vi "MainPhaseSpaceTracking.vi"() -> ()   [LabVIEW 2017]
uses:
  libowlsock.dll
panel:
  out "concatenated string":string
  in  "Button  Or UDP Sync":bool
  out "InvertVisualFbk":bool
  out "Imposed Time":i32
  out "Obj Initial Pos":dbl
  in  "Data Saveing Dir":string="Z:\\Toma_S\\DataProofs\\PhaseSpace\\"
  out "Shoulder":bool
  out "Elbow":bool
  out "refnum out":refnum<file>
  out "Data Filename":path
  out "Block":i32
  out "trial":u8
  out "Recording Switch":bool caption="Off       On"
  in  "Recording State":bool
  in  "UDP Sender Ip address":string="127.0.0.1"
  in  "ZeroTime":u32
  in  "ZeroFrame":i32
  out "Loop Time":u32
  out "Elapsed time (msec)":dbl
  out "Markers":dbl[](array[numeric])
  out "Frame Number":dbl
  in  "server address":string="192.168.0.101"
  out "connected\nto server?":bool
  out "Wrist":bool
  out "object":bool
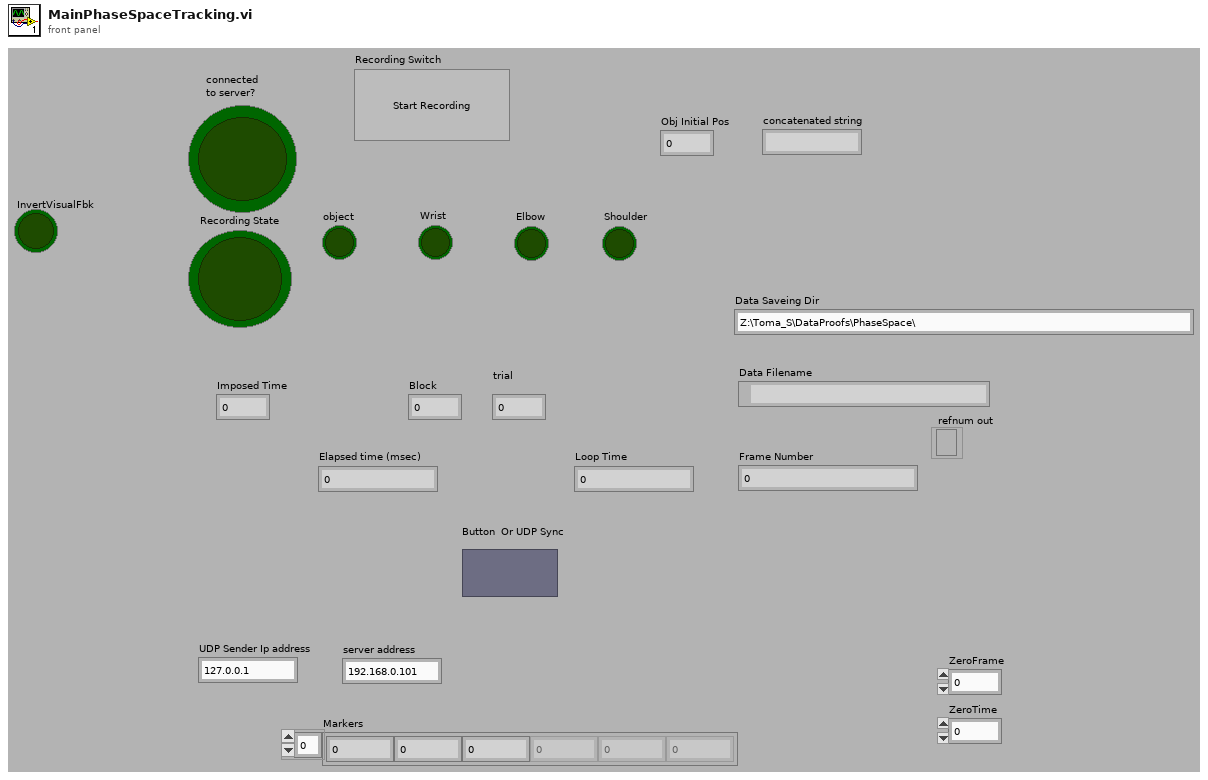
[diagram p1: front panel]
types:
  T1 = enum16{"open", "replace", "create", "open or create", "replace or create", "replace or create with confirmation"}
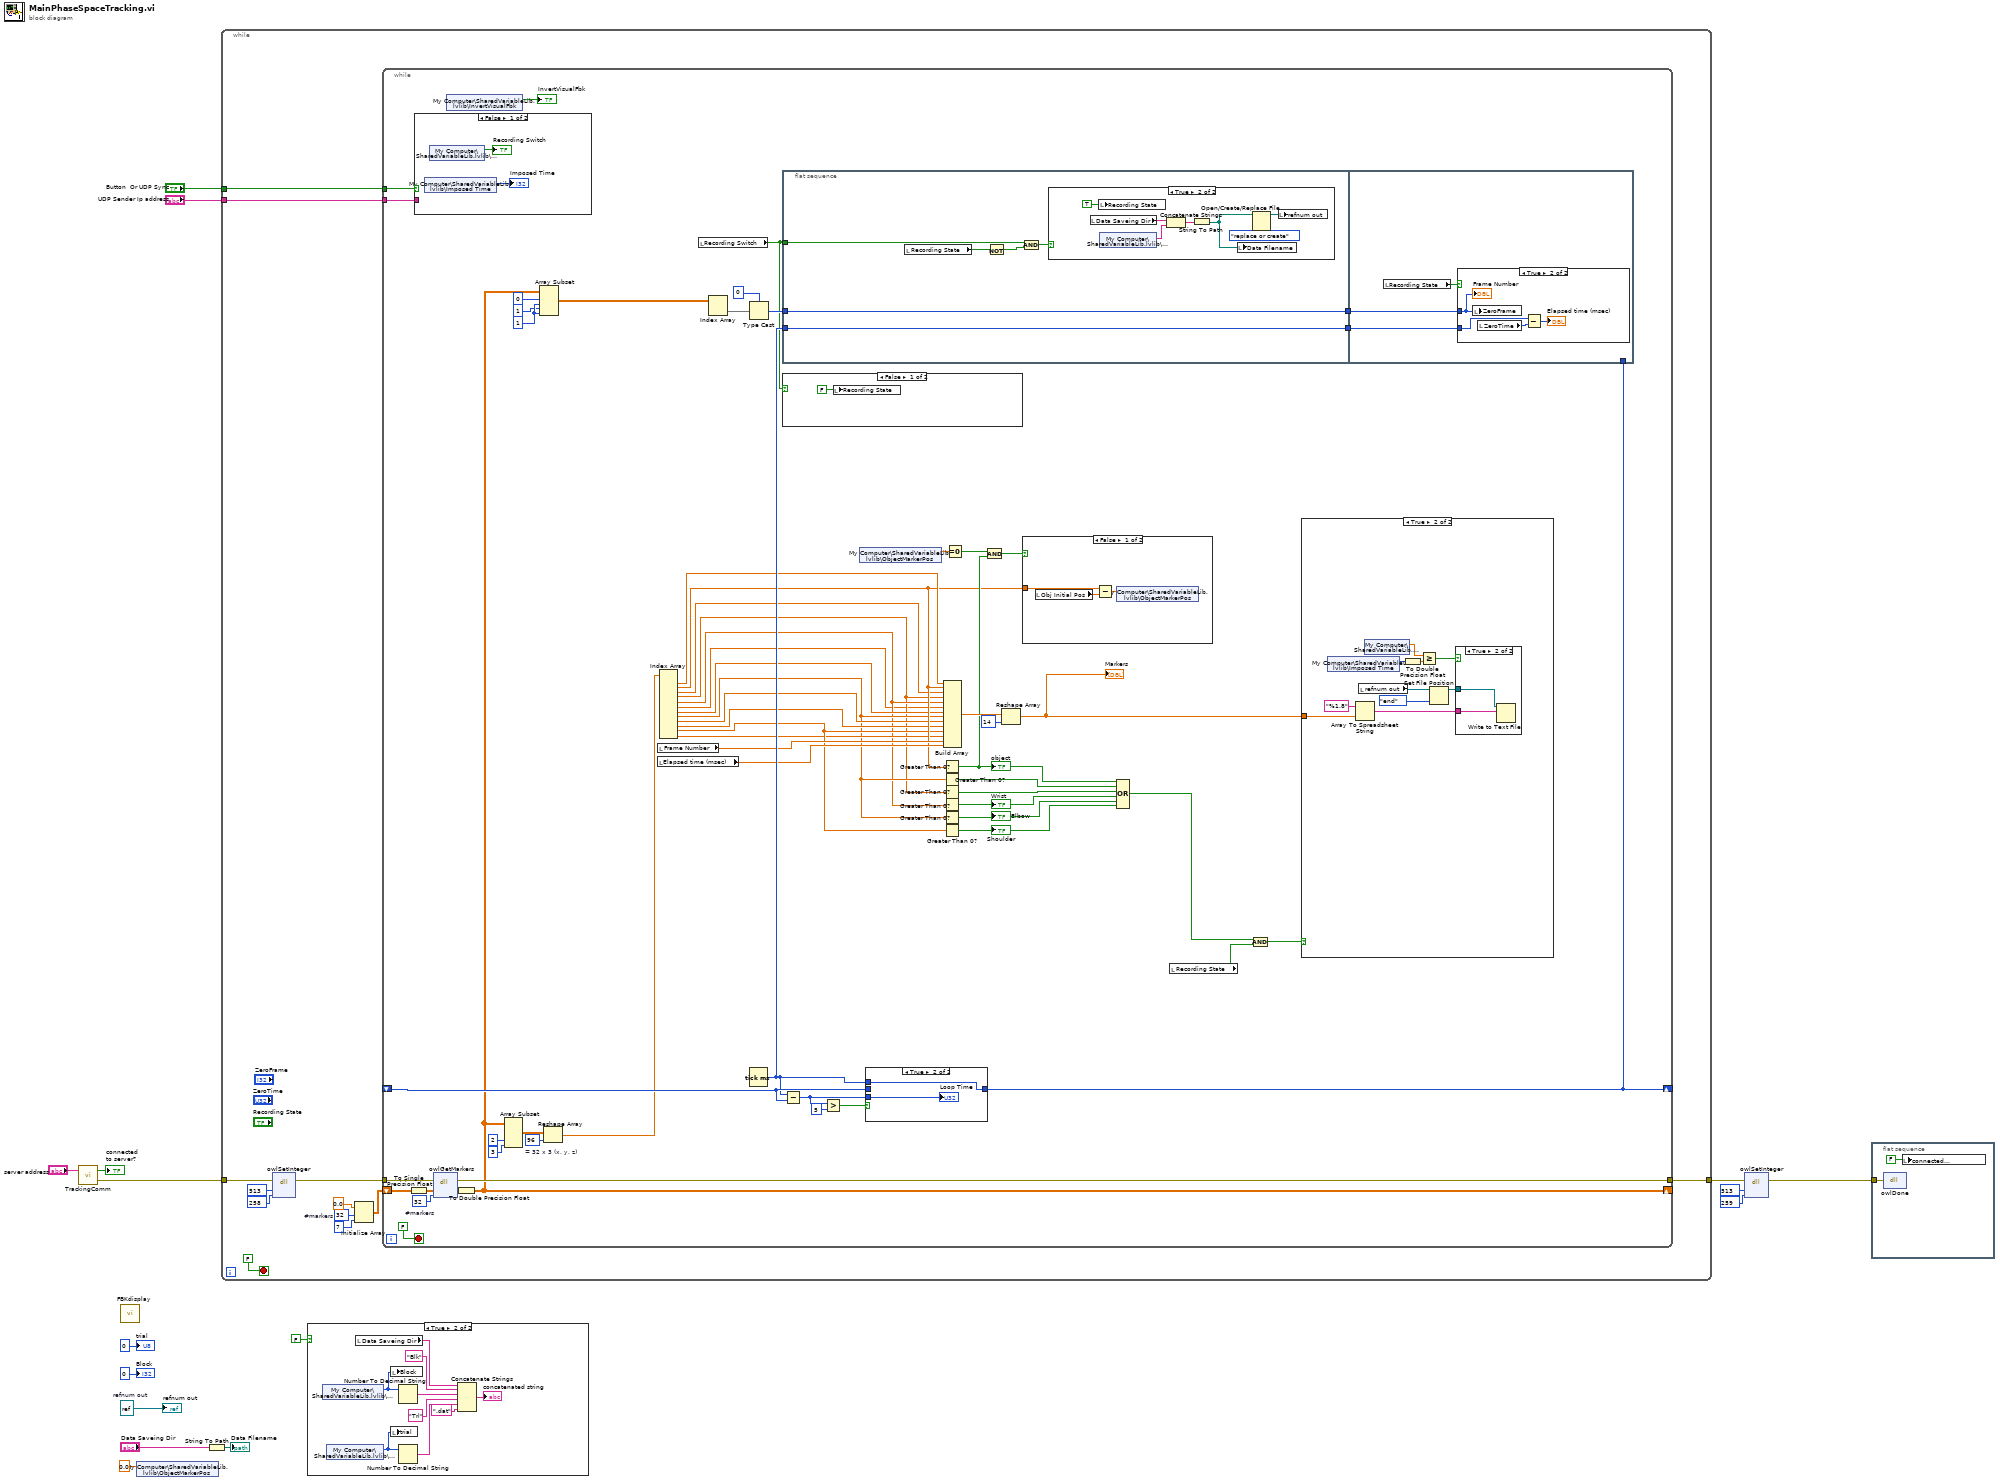
[diagram p0: block diagram]
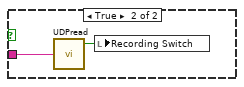
[diagram p2: hidden frame]
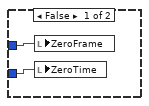
[diagram p4: hidden frame]
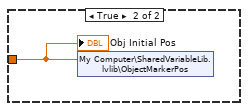
[diagram p7: hidden frame]
diagram:
  w8 = refnum<file> refnum  # refnum out
  n1 = call "TrackingComm.vi"("server address"="server address") -> ("error out"=w15:errorcluster, "connected to server?"=→"connected\nto server?":bool)  [unwired: 1 in]
  n2 = call "FBKdisplay.vi"() -> ()  [unwired: 10 in]
  n3 = shared-variable "My Computer\\SharedVariableLib.lvlib\\ObjectMarkerPos"(0.0) -> ()  [unwired: 1 in, 1 out]
  n4 = String To Path(string="Data Saveing Dir") -> (path=→"Data Filename":path)
  n5 = while {
    tunnel: w15 -> [w28]
    tunnel: [w20] -> w11
    tunnel: "UDP Sender Ip address" -> [w17]
    tunnel: "Button  Or UDP Sync" -> [w18]
    stop <- FALSE stop-if-true
    w27 = 32  # #markers
    n6 = dll-call lib="libowlsock.dll" fn="owlSetInteger"(error in=w28, "pname"=u16 513, "param"=u16 258) -> (error out=w21:errorcluster)  [unwired: 4 in, 2 out]
    n7 = Initialize Array(0.0, w27, 7) -> (w24:dbl[][])
    n8 = while {
      tunnel: [w79] -> w20
      shift-right: [w48] -> _
      shift-left: _ -> [w77]
      shift-right: [w43] -> _
      shift-left: w24 -> [w30]
      tunnel: w21 -> [w78]
      tunnel: w18 -> [w58]
      tunnel: w17 -> [w59]
      stop <- FALSE stop-if-true
      w65 = 1
      w86 = 96  # = 32 x 3 (x, y, z)
      w89 = u16 32  # #markers
      n9 = To Single Precision Float(number=w30) -> (single precision float=w29:sgl[][])
      n10 = case shown="False" w58 {
        tunnel: w59 -> [_ w93]
        frame False {
          n11 = shared-variable "My Computer\\SharedVariableLib.lvlib\\Imposed Time"() -> (→"Imposed Time":i32)  [unwired: 1 in, 1 out]
          n12 = shared-variable "My Computer\\SharedVariableLib.lvlib\\StartRec"() -> (→"Recording Switch":bool)  [unwired: 1 in, 1 out]
        }
        frame True {
          n13 = call "UDPread.vi"("Sender Ip address"=w93) -> ("recording Switch"=w92:bool)  [unwired: 2 out]
          n14 = local write "Recording Switch"(w92) -> ()
        }
      }
      n15 = dll-call lib="libowlsock.dll" fn="owlGetMarkers"(error in=w78, "markers"=w29, "count"=w89) -> (error out=w79:errorcluster, "markers"=w73:sgl[][])  [unwired: 3 in, 2 out]
      n16 = shared-variable "My Computer\\SharedVariableLib.lvlib\\InvertVisualFbk"() -> (→"InvertVisualFbk":bool)  [unwired: 1 in, 1 out]
      n17 = To Double Precision Float(number=w73) -> (double precision float=w43:dbl[][])
      n18 = Array Subset(array=w43, index (col)=2, length (col)=3) -> (w85:dbl[][])  [unwired: 2 in]
      n19 = Array Subset(array=w43, index (row)=0, length (row)=w65, index (col)=1, length (col)=w65) -> (w63:dbl[][])
      n20 = Reshape Array(w85, w86) -> (w49:dbl[])
      n21 = local read "Elapsed time (msec)"() -> (w45:dbl)
      n22 = local read "Frame Number"() -> (w46:dbl)
      n23 = Index Array(array=w49) -> (element #1=w71:dbl, element #2=w42:dbl, element #3=w41:dbl, element #4=w32:dbl, element #5=w33:dbl, element #6=w31:dbl, element #7=w40:dbl, element #8=w34:dbl, element #9=w39:dbl, element #10=w38:dbl, element #11=w37:dbl, element #12=w36:dbl)  [unwired: 12 in]
      n24 = local read "Recording Switch"() -> (w47:bool)
      n25 = Index Array(array=w63) -> (element=w62:dbl[])  [unwired: 2 in]
      n26 = Tick Count (ms)() -> (millisecond timer value=w76:u32)
      n27 = Type Cast(type=0, x=w62) -> (*(type *) &x=w60:i32)
      n28 = flat-sequence {
        tunnel: w60 -> [w96]
        tunnel: w47 -> [w98]
        tunnel: [w96] -> w67
        tunnel: w76 -> [w94]
        tunnel: [w94] -> w57
        tunnel: w67 -> [w108]
        tunnel: w48 -> [_]
        tunnel: w57 -> [w107]
        frame #0 {
          n29 = local read "Recording State"() -> (w95:bool)
          n30 = Not(x=w95) -> (.not. x?=w97:bool)
          n31 = And(x=w98, y=w97) -> (x .and. y?=w99:bool)
          n32 = case shown="True" w99 {
            frame False {
            }
            frame True {
              n33 = local read "Data Saveing Dir"() -> (w103:string)
              n34 = local write "Recording State"(TRUE) -> ()
              n35 = shared-variable "My Computer\\SharedVariableLib.lvlib\\FileName"() -> (w101:string)  [unwired: 1 in, 1 out]
              n36 = Concatenate Strings(w103, w101) -> (w102:string)
              n37 = String To Path(string=w102) -> (path=w105:path)
              n38 = local write "Data Filename"(w105) -> ()
              n39 = Open/Create/Replace File(file path (use dialog)=w105, operation (0:open)=T1."replace or create") -> (refnum out=w104:refnum<file>)  [unwired: 1 in, 5 out]
              n40 = local write "refnum out"(w104) -> ()
            }
          }
        }
        frame #1 {
          n41 = local read "Recording State"() -> (w109:bool)
          n42 = case shown="True" w109 {
            tunnel: w108 -> [w110 w112]
            tunnel: w107 -> [w111 w113]
            frame False {
              n43 = local write "ZeroFrame"(w110) -> ()
              n44 = local write "ZeroTime"(w111) -> ()
            }
            frame True {
              n45 = local write "ZeroFrame"(w112) -> ()
              n46 = local read "ZeroTime"() -> (w115:u32)
              n47 = Subtract(x=w113, y=w115) -> (x-y=→"Elapsed time (msec)":u32)
              "Frame Number" <- w112
            }
          }
        }
      }
      n48 = case shown="False" w47 {
        frame False {
          n49 = local write "Recording State"(FALSE) -> ()
        }
        frame True {
        }
      }
      n50 = Subtract(x=w76, y=w77) -> (x-y=w80:u32)
      n51 = Greater?(x=w80, y=u32 5) -> (0:w81:bool)
      n52 = shared-variable "My Computer\\SharedVariableLib.lvlib\\ObjectMarkerPos"() -> (w70:dbl)  [unwired: 1 in, 1 out]
      n53 = case shown="True" w81 {
        tunnel: w80 -> [_ w134]
        tunnel: [w133 w135] -> w48
        tunnel: w77 -> [w133 _]
        tunnel: w76 -> [_ w135]
        frame False {
        }
        frame True {
          "Loop Time" <- w134
        }
      }
      n54 = Build Array(w71, w42, w41, w32, w33, w31, w40, w34, w39, w38, w37, w36, w46, w45) -> (w84:dbl[])
      n55 = Greater Than 0?(x=w42) -> (x > 0?=w50:bool)
      "object" <- w50
      n56 = Greater Than 0?(x=w34) -> (x > 0?=w75:bool)
      n57 = Greater Than 0?(x=w32) -> (x > 0?=w74:bool)
      n58 = Greater Than 0?(x=w33) -> (x > 0?=w35:bool)
      "Wrist" <- w35
      n59 = Greater Than 0?(x=w34) -> (x > 0?=w44:bool)
      "Elbow" <- w44
      n60 = Greater Than 0?(x=w37) -> (x > 0?=w51:bool)
      "Shoulder" <- w51
      n61 = Equal To 0?(x=w70) -> (x = 0?=w69:bool)
      n62 = And(x=w69, y=w50) -> (x .and. y?=w68:bool)
      n63 = Reshape Array(w84, 14) -> (w53:dbl[])
      "Markers" <- w53
      n64 = case shown="False" w68 {
        tunnel: w42 -> [w130 w131]
        frame False {
          n65 = local read "Obj Initial Pos"() -> (w129:dbl)
          n66 = Subtract(x=w130, y=w129) -> (x-y=w128:dbl)
          n67 = shared-variable "My Computer\\SharedVariableLib.lvlib\\ObjectMarkerPos"(w128) -> ()  [unwired: 1 in, 1 out]
        }
        frame True {
          n68 = shared-variable "My Computer\\SharedVariableLib.lvlib\\ObjectMarkerPos"(w131) -> ()  [unwired: 1 in, 1 out]
          "Obj Initial Pos" <- w131
        }
      }
      n69 = Compound Arithmetic op=OR(w50, w75, w74, w35, w44, w51) -> (w56:bool)
      n70 = local read "Recording State"() -> (w55:bool)
      n71 = And(x=w56, y=w55) -> (x .and. y?=w54:bool)
      n72 = case shown="True" w54 {
        tunnel: w53 -> [_ w125]
        frame False {
        }
        frame True {
          n73 = shared-variable "My Computer\\SharedVariableLib.lvlib\\Imposed Time"() -> (w119:i32)  [unwired: 1 in, 1 out]
          n74 = Array To Spreadsheet String(array=w125, 3:"%1.8") -> (spreadsheet string=w124:string)  [unwired: 1 out]
          n75 = local read "refnum out"() -> (w118:refnum<file>)
          n76 = shared-variable "My Computer\\SharedVariableLib.lvlib\\Timer"() -> (w121:dbl)  [unwired: 1 in, 1 out]
          n77 = To Double Precision Float(number=w119) -> (double precision float=w116:dbl)
          n78 = Greater Or Equal?(x=w121, y=w116) -> (x >= y?=w120:bool)
          n79 = Set File Position(refnum=w118, from (0:start)=enum16{"start", "end", "current"}."end") -> (refnum out=w122:refnum<file>)  [unwired: 1 in, 2 out]
          n80 = case shown="True" w120 {
            tunnel: w124 -> [_ w127]
            tunnel: w122 -> [_ w126]
            frame False {
            }
            frame True {
              n81 = Write to Text File(file (use dialog)=w126, text=w127) -> ()  [unwired: 1 in, 4 out]
            }
          }
        }
      }
    }
  }
  n82 = case shown="True" FALSE {
    frame False {
    }
    frame True {
      n83 = shared-variable "My Computer\\SharedVariableLib.lvlib\\Block num"() -> (w137:i32)  [unwired: 1 in, 1 out]
      n84 = shared-variable "My Computer\\SharedVariableLib.lvlib\\Trial num"() -> (w138:i32)  [unwired: 1 in, 1 out]
      n85 = local read "Data Saveing Dir"() -> (w143:string)
      n86 = local write "Block"(w137) -> ()
      n87 = local write "trial"(w138) -> ()
      n88 = Number To Decimal String(number=w137) -> (decimal integer string=w144:string)  [unwired: 1 out]
      n89 = Number To Decimal String(number=w138) -> (decimal integer string=w140:string)  [unwired: 1 out]
      n90 = Concatenate Strings(w143, "Blk", w144, "Trl", w140, ".dat") -> (→"concatenated string":string)
    }
  }
  n91 = dll-call lib="libowlsock.dll" fn="owlSetInteger"(error in=w11, "pname"=u16 513, "param"=u16 259) -> (error out=w12:errorcluster)  [unwired: 4 in, 2 out]
  n92 = flat-sequence {
    tunnel: w12 -> [w146]
    frame #0 {
      n93 = dll-call lib="libowlsock.dll" fn="owlDone"(error in=w146) -> ()  [unwired: 2 in, 3 out]
      n94 = local write "connected\nto server?"(FALSE) -> ()
    }
  }
  "trial" <- u8 0
  "Block" <- 0
  "refnum out" <- w8
